vi "Swerve Autonomous.vi"(4 "Alternate Stop":bool, 6 "Robot Centric?":bool, 7 "Duration (sec)":dbl, 8 "Error In":errorcluster, 9 "Z":dbl, 10 "Y":dbl, 11 "X":dbl) -> (0 "Error Out":errorcluster)   [LabVIEW 2016]
uses:
  <vilib>/Rock Robotics/Network Tables/NT Read Number.vi
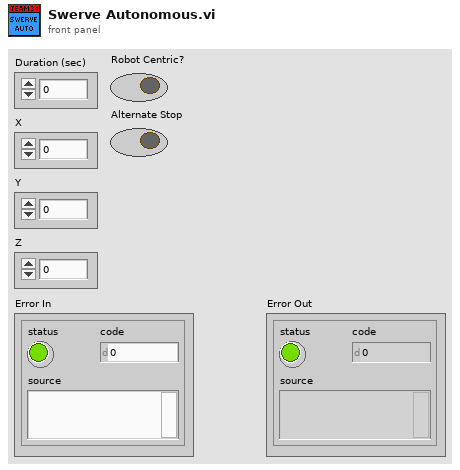
[diagram p1: front panel]
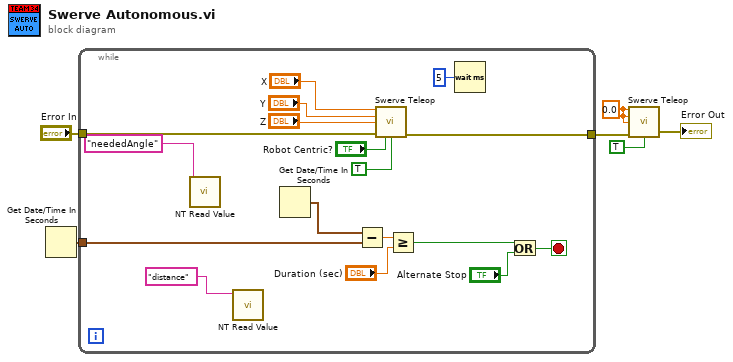
[diagram p0: block diagram]
diagram:
  w3 = 0.0 ("X")
  n1 = Get Date/Time In Seconds() -> (seconds since 1Jan1904=w6:timestamp)
  n2 = while {
    tunnel: w6 -> [w22]
    tunnel: "Error In" -> [w13]
    tunnel: [w12] -> w4
    stop <- w23 stop-if-true
    n3 = call-poly <vilib>:"NT Read Value.vi"("Name"="neededAngle") -> ()  [unwired: 9 in, 2 out]
    n4 = call-poly <vilib>:"NT Read Value.vi"("Name"="distance") -> ()  [unwired: 9 in, 2 out]
    n5 = Get Date/Time In Seconds() -> (seconds since 1Jan1904=w21:timestamp)
    n6 = Subtract(x=w21, y=w22) -> (x-y=w20:dbl)
    n7 = call "Swerve Teleop.vi"("X"="X", "Y"="Y", "Z"="Z", "Error In"=w13, "Robot Centric?"="Robot Centric?", "Autonomous?"=TRUE) -> ("Error Out"=w12:errorcluster)  [unwired: 5 in, 4 out]
    n8 = Greater Or Equal?(x=w20, y="Duration (sec)") -> (x >= y?=w9:bool)
    n9 = Wait (ms)(milliseconds to wait=u32 5) -> ()  [unwired: 1 out]
    n10 = Or(x=w9, y="Alternate Stop") -> (x .or. y?=w23:bool)
  }
  n11 = call "Swerve Teleop.vi"("X"=w3, "Y"=w3, "Z"=w3, "Error In"=w4, "Autonomous?"=TRUE) -> ("Error Out"=→"Error Out":errorcluster)  [unwired: 6 in, 4 out]
